vi "Cluster to C code.vi"(7 "indent code?":bool, 9 "typedef name":string, 10 "Cluster elements datatypes":string[](array[string]), 11 "Cluster elements names":string[](array[string])) -> (3 "C code":string)   [LabVIEW 2014]
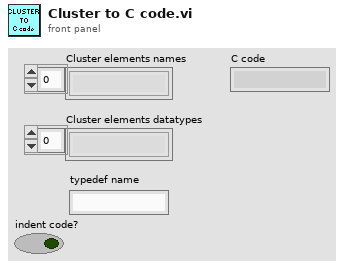
[diagram p1: front panel]
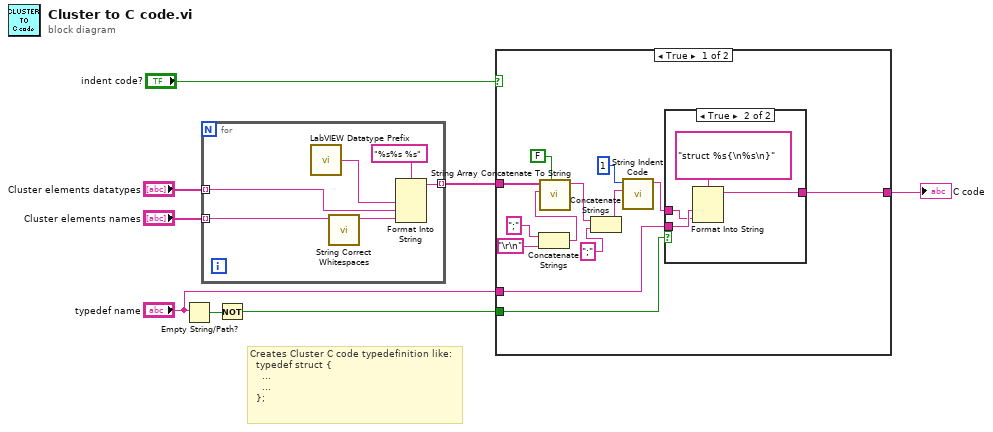
[diagram p0: block diagram]
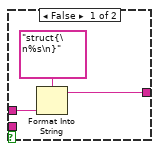
[diagram p2: hidden frame]
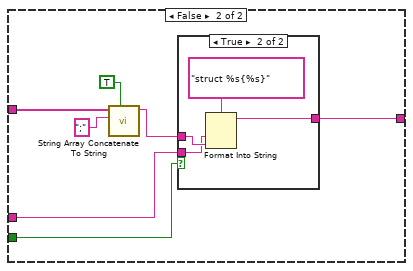
[diagram p3: hidden frame]
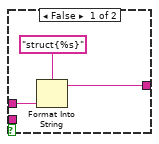
[diagram p4: hidden frame]
diagram:
  # "Creates Cluster C code typedefinition like:\n  typedef struct {\n    ...\n    ...\n  };"
  n1 = Empty String/Path?(string/path="typedef name") -> (empty?=w5:bool)
  n2 = for {
    tunnel: "Cluster elements names" -> [w9] mode=indexing
    tunnel: "Cluster elements datatypes" -> [w11] mode=indexing
    tunnel: [w12] -> w6 mode=indexing
    n3 = call "LabVIEW Datatype Prefix.vi"() -> ("datatype prefix"=w13:string)
    n4 = call "String Correct Whitespaces.vi"("String in"=w9) -> ("String out"=w10:string)  [unwired: 10 in]
    n5 = Format Into String(format string="%s%s %s", w13, w11, w10) -> (resulting string=w12:string)  [unwired: 2 in, 1 out]
  }
  n6 = Not(x=w5) -> (.not. x?=w4:bool)
  n7 = case shown="True" "indent code?" {
    tunnel: w6 -> [w27 w40]
    tunnel: w4 -> [w23 w38]
    tunnel: "typedef name" -> [w22 w37]
    tunnel: [w21 w36] -> w2
    frame True {
      n8 = Concatenate Strings(";" ("format string"), "\r\n") -> (w18:string)
      n9 = call "String Array Concatenate To String.vi"("insert last delimiter?"=FALSE, "Delimiter char"=w18, "Array String In"=w27) -> ("String"=w17:string)  [unwired: 8 in]
      n10 = Concatenate Strings(w17, ";" ("format string")) -> (w16:string)
      n11 = call "String Indent Code.vi"("complete code"=w16, "actual nested level"=1) -> ("indented code"=w19:string)  [unwired: 9 in]
      n12 = case shown="True" w23 {
        tunnel: [w30 w34] -> w21
        tunnel: w22 -> [_ w32]
        tunnel: w19 -> [w28 w31]
        frame False {
          n13 = Format Into String(format string="struct{\n%s\n}", w28) -> (resulting string=w30:string)  [unwired: 2 in, 1 out]
        }
        frame True {
          n14 = Format Into String(format string="struct %s{\n%s\n}", w32, w31) -> (resulting string=w34:string)  [unwired: 2 in, 1 out]
        }
      }
    }
    frame False {
      n15 = call "String Array Concatenate To String.vi"("insert last delimiter?"=TRUE, "Delimiter char"=";" ("format string"), "Array String In"=w40) -> ("String"=w41:string)  [unwired: 8 in]
      n16 = case shown="True" w38 {
        tunnel: [w44 w48] -> w36
        tunnel: w41 -> [w43 w46]
        tunnel: w37 -> [_ w45]
        frame False {
          n17 = Format Into String(format string="struct{%s}", w43) -> (resulting string=w44:string)  [unwired: 2 in, 1 out]
        }
        frame True {
          n18 = Format Into String(format string="struct %s{%s}", w45, w46) -> (resulting string=w48:string)  [unwired: 2 in, 1 out]
        }
      }
    }
  }
  "C code" <- w2
